vi "jsonParseDbl.vi"(8 "error in (no error)":errorcluster, 9 "default":dbl, 10 "path":string, 11 "d in":i64) -> (0 "error out":errorcluster, 2 "value":dbl, 3 "d out":i64)   [LabVIEW 2015, in "rapidjson wrapper.lvlib"]
uses:
  rapidjson wrapper.lvlib
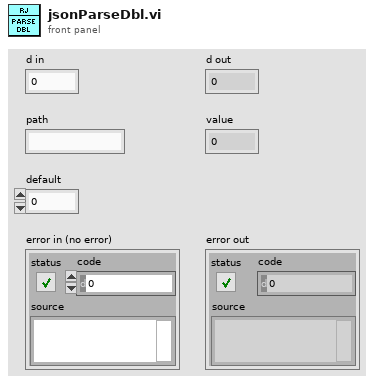
[diagram p1: front panel]
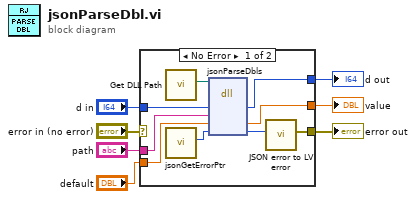
[diagram p0: block diagram]
diagram:
  n1 = case shown="No Error" "error in (no error)" {
    selector: "error in (no error)" -> [_ w19]
    tunnel: [w14 w19] -> w7
    tunnel: [w11 w18] -> w5
    tunnel: "default" -> [w12 w18]
    tunnel: [w10 w17] -> w3
    tunnel: "d in" -> [w9 w17]
    tunnel: "path" -> [w8 _]
    frame No Error {
      n2 = call "Get DLL Path.vi"() -> ("Path"=w16:path)  [unwired: 11 in]
      n3 = call "jsonGetErrorPtr.vi"() -> ("return type"=w13:i64)  [unwired: 10 in, 1 out]
      n4 = dll-call lib="C:/Users/tblair/Documents/Git Projects/LVrapidjson core/lvrjs/Debug/lvrjs.dll" fn="jsonParseDbls"(path in=w16, "d"=w9, "path"=w8, "default"=w12, "jsonError"=w13) -> ("d"=w10:i64, "default"=w11:dbl, "jsonError"=w15:i64)  [unwired: 4 in, 2 out]
      n5 = call "JSON error to LV error.vi"("jsonError"=w15) -> ("error out"=w14:errorcluster)  [unwired: 10 in]
    }
    frame Error {
    }
  }
  "error out" <- w7
  "value" <- w5
  "d out" <- w3
